vi "Control motors simuntaniously.vi"() -> ()   [LabVIEW 2016]
uses:
  Motor controllers.vi
  <vilib>/CANopenLib/CANOPEN.llb/CANopen SDO Create.vi
  Set mode of operation.vi
  Set control mode.vi
  Set into drive mode.vi
  Get mode of operation.vi
  Set target speed.vi
  <vilib>/CANopenLib/CANOPEN.llb/CANopen SDO Close.vi
panel:
  out "Error 2":errorcluster
  in  "Motor Speed 2":i32(knob) scale=0.0..1500.0
  out "completion code 9":u32
  out "completion code 8":u32
  out "Mode of operation 2":i8(ring) items=["Induction VF – testing purposes only"=-5, "Aligning rotor position"=-4, "Current stepper – testing purposes only "=-3, "Voltage stepper – testing purposes only"=-2, "Voltage constant angle – testing purposes only"=-1, "No mode"=0, "Cyclic sync position"=8, "Cyclic sync velocity"=9, "Cyclic sync torque"=10]
  out "Mode of operation":i8(ring) items=["Induction VF – testing purposes only"=-5, "Aligning rotor position"=-4, "Current stepper – testing purposes only "=-3, "Voltage stepper – testing purposes only"=-2, "Voltage constant angle – testing purposes only"=-1, "No mode"=0, "Cyclic sync position"=8, "Cyclic sync velocity"=9, "Cyclic sync torque"=10]
  in  "Stop Button":bool
  out "Error":errorcluster
  in  "Motor Speed":i32(knob) scale=0.0..1500.0
  out "completion code 7":u32
  out "completion code 6":u32
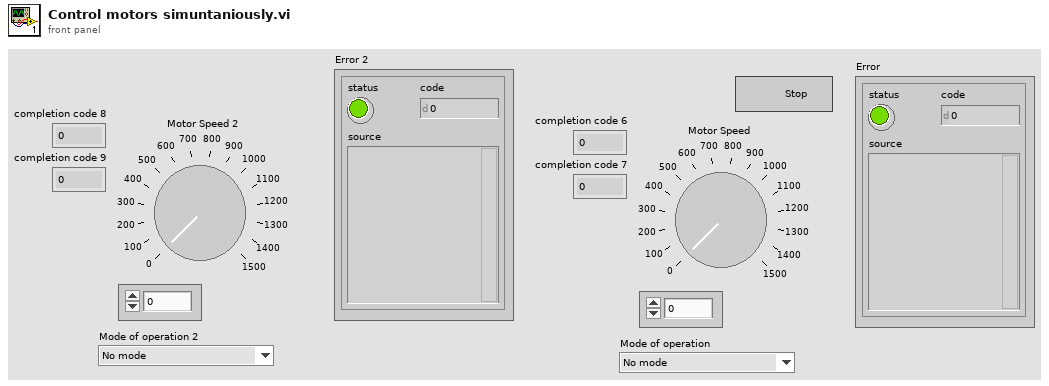
[diagram p1: front panel]
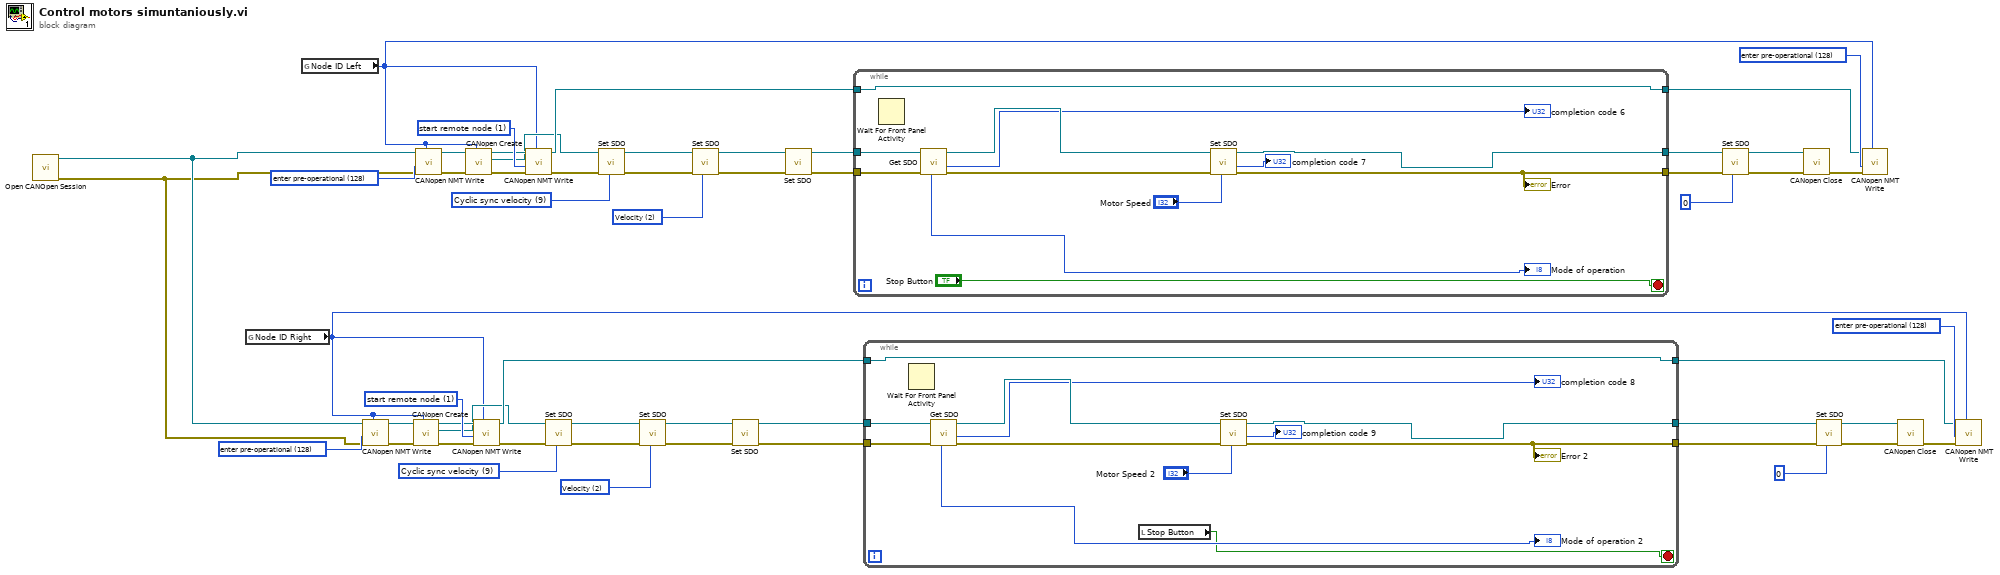
[diagram p0: block diagram]
diagram:
  w3 = u16 128 items=["start remote node"=1, "stop remote node"=2, "enter pre-operational"=128, "reset node"=129, "reset communication"=130] ("command")
  w11 = u16 1 items=["start remote node"=1, "stop remote node"=2, "enter pre-operational"=128, "reset node"=129, "reset communication"=130] ("command")
  w16 = i8 9 items=["Induction VF – testing purposes only"=-5, "Aligning rotor position"=-4, "Current stepper – testing purposes only "=-3, "Voltage stepper – testing purposes only"=-2, "Voltage constant angle – testing purposes only"=-1, "No mode"=0, "Cyclic sync position"=8, "Cyclic sync velocity"=9, "Cyclic sync torque"=10] ("Mode of operation")
  w21 = u8 2 items=["Velocity"=2, "Torque"=1] ("Control Mode")
  w27 = u16 128 items=["start remote node"=1, "stop remote node"=2, "enter pre-operational"=128, "reset node"=129, "reset communication"=130] ("command")
  w29 = u16 128 items=["start remote node"=1, "stop remote node"=2, "enter pre-operational"=128, "reset node"=129, "reset communication"=130] ("command")
  w37 = u16 1 items=["start remote node"=1, "stop remote node"=2, "enter pre-operational"=128, "reset node"=129, "reset communication"=130] ("command")
  w42 = i8 9 items=["Induction VF – testing purposes only"=-5, "Aligning rotor position"=-4, "Current stepper – testing purposes only "=-3, "Voltage stepper – testing purposes only"=-2, "Voltage constant angle – testing purposes only"=-1, "No mode"=0, "Cyclic sync position"=8, "Cyclic sync velocity"=9, "Cyclic sync torque"=10] ("Mode of operation")
  w47 = u8 2 items=["Velocity"=2, "Torque"=1] ("Control Mode")
  w53 = u16 128 items=["start remote node"=1, "stop remote node"=2, "enter pre-operational"=128, "reset node"=129, "reset communication"=130] ("command")
  n1 = call "Open CANOpen Session.vi"() -> ("error out"=w1:errorcluster, "interface object out"=w2:refnum<k20>)  [unwired: 10 in]
  n2 = global read "Motor controllers.vi" "Node ID Right"() -> (w4:u8)
  n3 = global read "Motor controllers.vi" "Node ID Left"() -> (w30:u8)
  n4 = call <vilib>:"CANopen NMT Write.vi"("node-ID (0)"=w4, "error in (no error)"=w1, "command"=w3, "interface object in"=w2) -> ("error out"=w6:errorcluster, "interface object out"=w5:refnum<k20>)  [unwired: 6 in]
  n5 = call-poly <vilib>:"CANopen Create.vi"("node-ID"=w4, "error in (no error)"=w6, "interface object in"=w5) -> ("error out"=w8:errorcluster, "SDO object out"=w9:refnum<k20>, "interface object out"=w10:refnum<k20>)  [unwired: 6 in]
  n6 = call <vilib>:"CANopen NMT Write.vi"("node-ID (0)"=w30, "error in (no error)"=w1, "command"=w29, "interface object in"=w2) -> ("error out"=w32:errorcluster, "interface object out"=w31:refnum<k20>)  [unwired: 6 in]
  n7 = call-poly <vilib>:"CANopen Create.vi"("node-ID"=w30, "error in (no error)"=w32, "interface object in"=w31) -> ("error out"=w34:errorcluster, "SDO object out"=w35:refnum<k20>, "interface object out"=w36:refnum<k20>)  [unwired: 6 in]
  n8 = call <vilib>:"CANopen NMT Write.vi"("node-ID (0)"=w4, "error in (no error)"=w8, "command"=w11, "interface object in"=w10) -> ("error out"=w12:errorcluster, "interface object out"=w13:refnum<k20>)  [unwired: 6 in]
  n9 = call <vilib>:"CANopen NMT Write.vi"("node-ID (0)"=w30, "error in (no error)"=w34, "command"=w37, "interface object in"=w36) -> ("error out"=w38:errorcluster, "interface object out"=w39:refnum<k20>)  [unwired: 6 in]
  n10 = call-poly "Set SDO.vi"("Mode of operation"=w16, "error in (no error)"=w12, "SDO object in"=w9) -> ("error out"=w19:errorcluster, "SDO object out"=w20:refnum<k20>)  [unwired: 6 in, 1 out]
  n11 = call-poly "Set SDO.vi"("Mode of operation"=w42, "error in (no error)"=w38, "SDO object in"=w35) -> ("error out"=w45:errorcluster, "SDO object out"=w46:refnum<k20>)  [unwired: 6 in, 1 out]
  n12 = call-poly "Set SDO.vi"("Control Mode"=w21, "error in (no error)"=w19, "SDO object in"=w20) -> ("error out"=w17:errorcluster, "SDO object out"=w18:refnum<k20>)  [unwired: 6 in, 1 out]
  n13 = call-poly "Set SDO.vi"("Control Mode"=w47, "error in (no error)"=w45, "SDO object in"=w46) -> ("error out"=w43:errorcluster, "SDO object out"=w44:refnum<k20>)  [unwired: 6 in, 1 out]
  n14 = call-poly "Set SDO.vi"("error in (no error)"=w17, "SDO object in"=w18) -> ("error out"=w14:errorcluster, "SDO object out"=w15:refnum<k20>)  [unwired: 8 in]
  n15 = call-poly "Set SDO.vi"("error in (no error)"=w43, "SDO object in"=w44) -> ("error out"=w40:errorcluster, "SDO object out"=w41:refnum<k20>)  [unwired: 8 in]
  n16 = while {
    tunnel: [w65] -> w52
    tunnel: [w63] -> w51
    tunnel: w39 -> [w64]
    tunnel: [w64] -> w33
    tunnel: w41 -> [w60]
    tunnel: w40 -> [w59]
    stop <- "Stop Button" stop-if-true
    n17 = Wait For Front Panel Activity() -> ()  [unwired: 3 in, 1 out]
    n18 = call-poly "Get SDO.vi"("error in (no error)"=w59, "SDO object in"=w60) -> ("error out"=w61:errorcluster, "completion code"=→"completion code 6":u32, "SDO object out"=w62:refnum<k20>, "Mode of operation"=→"Mode of operation":i8)  [unwired: 6 in]
    n19 = call-poly "Set SDO.vi"("Speed"="Motor Speed", "error in (no error)"=w61, "SDO object in"=w62) -> ("error out"=w63:errorcluster, "completion code"=→"completion code 7":u32, "SDO object out"=w65:refnum<k20>)  [unwired: 6 in]
    "Error" <- w63
  }
  n20 = while {
    tunnel: [w78] -> w26
    tunnel: [w76] -> w25
    tunnel: w13 -> [w77]
    tunnel: [w77] -> w7
    tunnel: w15 -> [w73]
    tunnel: w14 -> [w72]
    stop <- w67 stop-if-true
    n21 = Wait For Front Panel Activity() -> ()  [unwired: 3 in, 1 out]
    n22 = call-poly "Get SDO.vi"("error in (no error)"=w72, "SDO object in"=w73) -> ("error out"=w74:errorcluster, "completion code"=→"completion code 8":u32, "SDO object out"=w75:refnum<k20>, "Mode of operation"=→"Mode of operation 2":i8)  [unwired: 6 in]
    n23 = local read "Stop Button"() -> (w67:bool)
    n24 = call-poly "Set SDO.vi"("Speed"="Motor Speed 2", "error in (no error)"=w74, "SDO object in"=w75) -> ("error out"=w76:errorcluster, "completion code"=→"completion code 9":u32, "SDO object out"=w78:refnum<k20>)  [unwired: 6 in]
    "Error 2" <- w76
  }
  n25 = call-poly "Set SDO.vi"("Speed"=0, "error in (no error)"=w51, "SDO object in"=w52) -> ("error out"=w50:errorcluster, "SDO object out"=w49:refnum<k20>)  [unwired: 6 in, 1 out]
  n26 = call-poly <vilib>:"CANopen Close.vi"("error in (no error)"=w50, "SDO object in"=w49) -> ("error out"=w48:errorcluster)  [unwired: 9 in]
  n27 = call-poly "Set SDO.vi"("Speed"=0, "error in (no error)"=w25, "SDO object in"=w26) -> ("error out"=w24:errorcluster, "SDO object out"=w23:refnum<k20>)  [unwired: 6 in, 1 out]
  n28 = call <vilib>:"CANopen NMT Write.vi"("node-ID (0)"=w30, "error in (no error)"=w48, "command"=w53, "interface object in"=w33) -> ()  [unwired: 6 in, 2 out]
  n29 = call-poly <vilib>:"CANopen Close.vi"("error in (no error)"=w24, "SDO object in"=w23) -> ("error out"=w22:errorcluster)  [unwired: 9 in]
  n30 = call <vilib>:"CANopen NMT Write.vi"("node-ID (0)"=w4, "error in (no error)"=w22, "command"=w27, "interface object in"=w7) -> ()  [unwired: 6 in, 2 out]
